vi "Acquisition & Generation (Init Memory) test UI.vi"() -> ()   [LabVIEW 2014]
uses:
  <vilib>/rvi/interface/RandomDataEmulation/nirviRandomDataOpen.vi
  <vilib>/rvi/interface/common/niFpgaCacheSessionInfoDynamic.vi
  <vilib>/rvi/interface/common/niFpgaWaitOnOcc.vi
  <vilib>/Utility/error.llb/Error Cluster From Error Code.vi
  <vilib>/FPGAPlugInAG/Dynamic/niLvFpga_Run_Dynamic.vi
  <vilib>/rvi/errors/niLvFpgaAdjustHostInterfaceError.vi
  <vilib>/FPGAPlugInAG/Dynamic/niLvFpga_Close_Dynamic.vi
  <vilib>/rvi/interface/nirviOpenFPGA/nirviOpenFPGA.xnode
  FPGA Target/Test VIs/Acquisition & Generation (Init Memory) test.vi
  <vilib>/rvi/interface/nirviMethod/nirviMethod.xnode
  <vilib>/rvi/interface/nirviCloseFPGA/nirviCloseFPGA.xnode
  <vilib>/FPGAPlugInAG/Dynamic/niLvFpga_ConfigureFifo_Dynamic.vi
  <vilib>/rvi/errors/niLvFpgaMergeErrorWithErrorCode.vi
  <vilib>/FPGAPlugInAG/Dynamic/niLvFpga_StartFifo_Dynamic.vi
  <vilib>/FPGAPlugInAG/Dynamic/niLvFpga_ReadFifo_Dynamic.vi
panel:
  out "Signal write on memory":dbl[](graph)
  in  "Single acquisition (F)":bool
  out "Write memory complete":bool
  out "Acquired Signal":dbl[](graph)
  # "Continuous acquisition (T)"
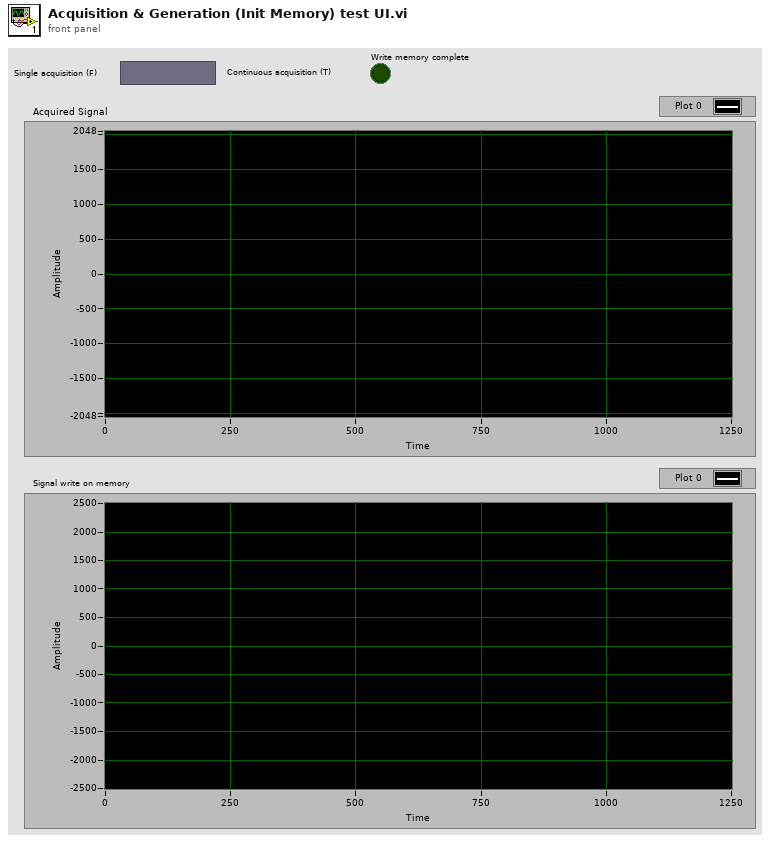
[diagram p1: front panel]
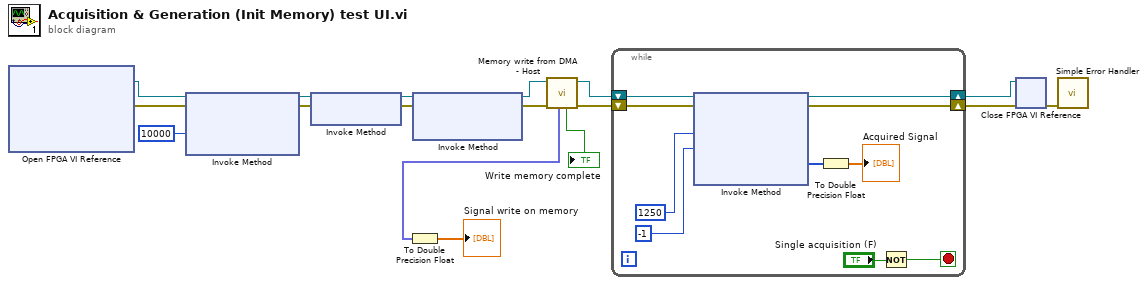
[diagram p0: block diagram]
diagram:
  n1 = xnode "Open FPGA VI Reference"() -> ("FPGA VI Reference Out"=w17:refnum<k20>, "error out"=w16:errorcluster)  [unwired: 2 in]
  n2 = xnode "Invoke Method"("FPGA VI Reference In"=w17, "error in"=w16, "Requested Depth"=u32 10000) -> ("FPGA VI Reference Out"=w13:refnum<k20>, "error out"=w14:errorcluster)  [unwired: 1 out]
  n3 = xnode "Invoke Method"("FPGA VI Reference In"=w13, "error in"=w14) -> ("FPGA VI Reference Out"=w11:refnum<k20>, "error out"=w12:errorcluster)
  n4 = xnode "Invoke Method"("FPGA VI Reference In"=w11, "error in"=w12) -> ("FPGA VI Reference Out"=w7:refnum<k20>, "error out"=w5:errorcluster)  [unwired: 1 in]
  n5 = call "Memory write from DMA - Host.vi"("error in"=w5, "FPGA VI Reference In"=w7) -> ("error out"=w4:errorcluster, "FPGA VI Reference Out"=w6:refnum<k20>, "Write memory complete"=→"Write memory complete":bool, "FXP Init Data Out"=w1:fxp<+/-,12,12>[])  [unwired: 6 in]
  n6 = To Double Precision Float(number=w1) -> (double precision float=→"Signal write on memory":dbl[])
  n7 = while {
    shift-right: [w27] -> w9
    shift-left: w6 -> [w22]
    shift-right: [w26] -> w8
    shift-left: w4 -> [w21]
    stop <- w18 stop-if-true
    n8 = xnode "Invoke Method"("FPGA VI Reference In"=w22, "error in"=w21, "Number of Elements"=u32 1250, "Timeout (ms)"=-1) -> ("FPGA VI Reference Out"=w27:refnum<k20>, "error out"=w26:errorcluster, "Data"=w24:i16[])  [unwired: 1 out]
    n9 = To Double Precision Float(number=w24) -> (double precision float=→"Acquired Signal":dbl[])
    n10 = Not(x="Single acquisition (F)") -> (.not. x?=w18:bool)
  }
  n11 = xnode "Close FPGA VI Reference"("FPGA VI Reference In"=w9, "error in"=w8) -> ("error out"=w10:errorcluster)
  n12 = call <vilib>:"Simple Error Handler.vi"("error in (no error)"=w10) -> ()  [unwired: 4 in, 5 out]
